vi "Configure PRACH Limit Frequency Error.vi"(7 "Limit Value (0.1)":dbl=0.1 format="%^.3e", 8 "error in (no error)":errorcluster, 9 "Limit Check Enabled (Value)":i32(ring)=2 items=["Off", "On", "Value"], 10 "Instance (1)":T1=1, 11 "VISA resource name":refnum<visa-resource-name>) -> (0 "error out":errorcluster, 3 "VISA resource name out":refnum<visa-resource-name>)   [LabVIEW 2020, in "Rohde&Schwarz CMWXP NR FR1 Measurement.lvlib"]
doc: "Defines an upper limit for the carrier frequency error.\n\nAttributes:\nRSCMWXPNRFR1M_ATTR_PRACH_LIMIT_FREQUENCY_ERROR_ENABLED\nRSCMWXPNRFR1M_ATTR_PRACH_LIMIT_FREQUENCY_ERROR\n\nRemote-control command:\nCONFigure:NRSub:MEAS<i>:PRACh:LIMit:FERRor"
uses:
  <instrlib>/Rohde&Schwarz CMWXP NR FR1 Measurement/Rohde&Schwarz CMWXP NR FR1 Measurement.lvlib
  <instrlib>/Rohde&Schwarz CMWXP NR FR1 Measurement/Private/_Instance.ctl
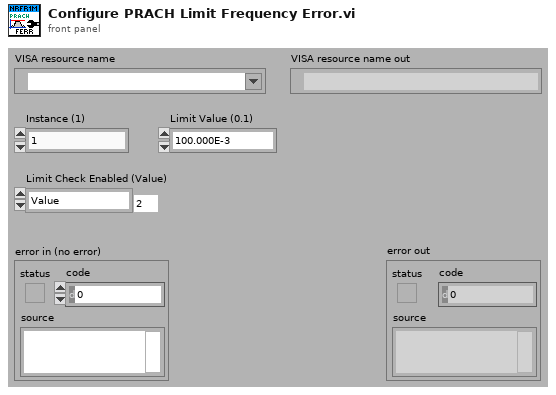
[diagram p1: front panel]
types:
  T1 = typedef "Rohde&Schwarz CMWXP NR FR1 Measurement.lvlib/_Instance.ctl" = i32
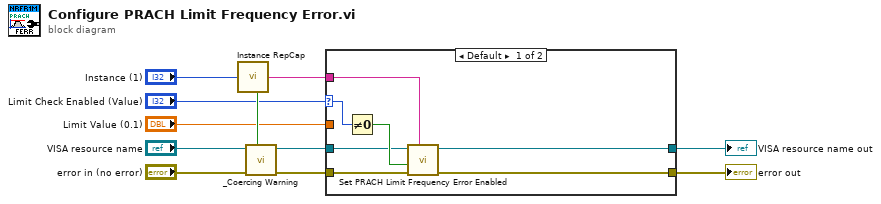
[diagram p0: block diagram]
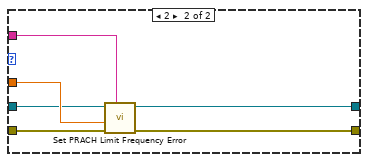
[diagram p2: hidden frame]
diagram:
  n1 = call <instrlib>:"Instance RepCap.vi"("Instance In"="Instance (1)") -> ("In Range?"=w8:bool, "RepCap Identifier Out"=w1:string)  [unwired: 1 in]
  n2 = call <instrlib>:"_Coercing Warning.vi"("In Range?"=w8, "error in (no error)"="error in (no error)", "VISA resource name"="VISA resource name") -> ("error out"=w5:errorcluster, "VISA resource name out"=w4:refnum<visa-resource-name>)  [unwired: 7 in]
  n3 = case shown="Default" "Limit Check Enabled (Value)" {
    selector: "Limit Check Enabled (Value)" -> [w12 _]
    tunnel: "Limit Value (0.1)" -> [_ w24]
    tunnel: [w17 w22] -> w3
    tunnel: [w16 w23] -> w2
    tunnel: w5 -> [w15 w21]
    tunnel: w4 -> [w14 w20]
    tunnel: w1 -> [w13 w19]
    frame Default {
      n4 = Not Equal To 0?(x=w12) -> (x != 0?=w18:bool)
      n5 = call "Set PRACH Limit Frequency Error Enabled"("Repeated Capabilities"=w13, "error in (no error)"=w15, "PRACH Limit Frequency Error Enabled (OFF)"=w18, "instrument handle"=w14) -> ("error out"=w17:errorcluster, "instrument handle out"=w16:refnum<visa-resource-name>)  [unwired: 6 in]
    }
    frame 2 {
      n6 = call "Set PRACH Limit Frequency Error"("Repeated Capabilities"=w19, "error in (no error)"=w21, "PRACH Limit Frequency Error (0.0)"=w24, "instrument handle"=w20) -> ("error out"=w22:errorcluster, "instrument handle out"=w23:refnum<visa-resource-name>)  [unwired: 6 in]
    }
  }
  "error out" <- w3
  "VISA resource name out" <- w2
